vi "Main.vi"(11 "Module Admin":refnum<class "Delacor_lib_QMH_Module Admin.lvclass">) -> ()   [LabVIEW 2014, in "get_data_mapper.lvlib"]
doc: "This template is based off of the Queued Message Handler design pattern and the Queued Message Handler project template that ships with LabVIEW.\n\nThe main difference is that the queue is private to this module and communication between modules is performed via Broadcast and Request events.\n\nRequest events are wrapped in public API methods and are handled in the Event Handling Loop (EHL) of this VI. Any module can register for Broadcast events sent by this module. The EHL generates messages based on user interface actions.\n\nThe Message Handling Loop (MHL) processes messages generated by the EHL, or by other messages. The messages are string values, so new messages can be added easily to the Message Cases case structure in the MHL. Each message cluster can also provide an optional value for Message Data, which is a variant that can be converted to whatever message-specific data is required.\n_____\nBased on DQMH Project Template 6.0.0.91."
uses:
  get_data_mapper.lvlib
  <vilib>/Delacor/Delacor QMH/Libraries/Module Admin_class/Delacor_lib_QMH_Module Admin.lvclass
  Module Data--cluster.ctl
  <vilib>/Delacor/Delacor QMH/Libraries/Message Queue_class/Delacor_lib_QMH_Message Queue.lvclass/Delacor_lib_QMH_Message Queue.ctl
  Stop Argument--cluster.ctl
  <vilib>/Delacor/Delacor QMH/Libraries/Module Admin_class/Delacor_lib_QMH_Module Admin.lvclass/Delacor_lib_QMH_Module Admin.ctl
  <vilib>/Utility/miscctls.llb/LVPointTypeDef.ctl
  <vilib>/Delacor/Delacor QMH/Libraries/Message Queue_class/Delacor_lib_QMH_Enqueue Message (Single).vi
  <vilib>/Delacor/Delacor QMH/Libraries/Module Admin_class/Delacor_lib_QMH_Get External Launch.vi
  <vilib>/Utility/error.llb/Error Cluster From Error Code.vi
  <vilib>/ErrorRing/Error Ring.xnode
  <vilib>/Delacor/Delacor QMH/Libraries/Message Queue_class/Delacor_lib_QMH_Message Queue.lvclass
panel:
  out "Data names":string[](array[string])=["Tc01", "Tc02"]
  in  "Data names Input":string[](array[string])=["Loop_number ", "Error_number", "Error_number_2", "DI_no1", "Flow"]
  in  "Update Names":bool
  out "Data out string":string="{\"Tc01\":1.000000,\"Tc02\":2.000000}"
  in  "Data sources":refnum<k21>[](array[refnum])=["ni.var.psp://my computer/Test Data/testdata1"]
  out "Data Out":dbl[](array[numeric])=[1.0, 2.0]
  out "error out":errorcluster
  out "Status":string="Initial Message"
  in  "Simulate MHL Error":bool
  in  "Simulate EHL Error":bool
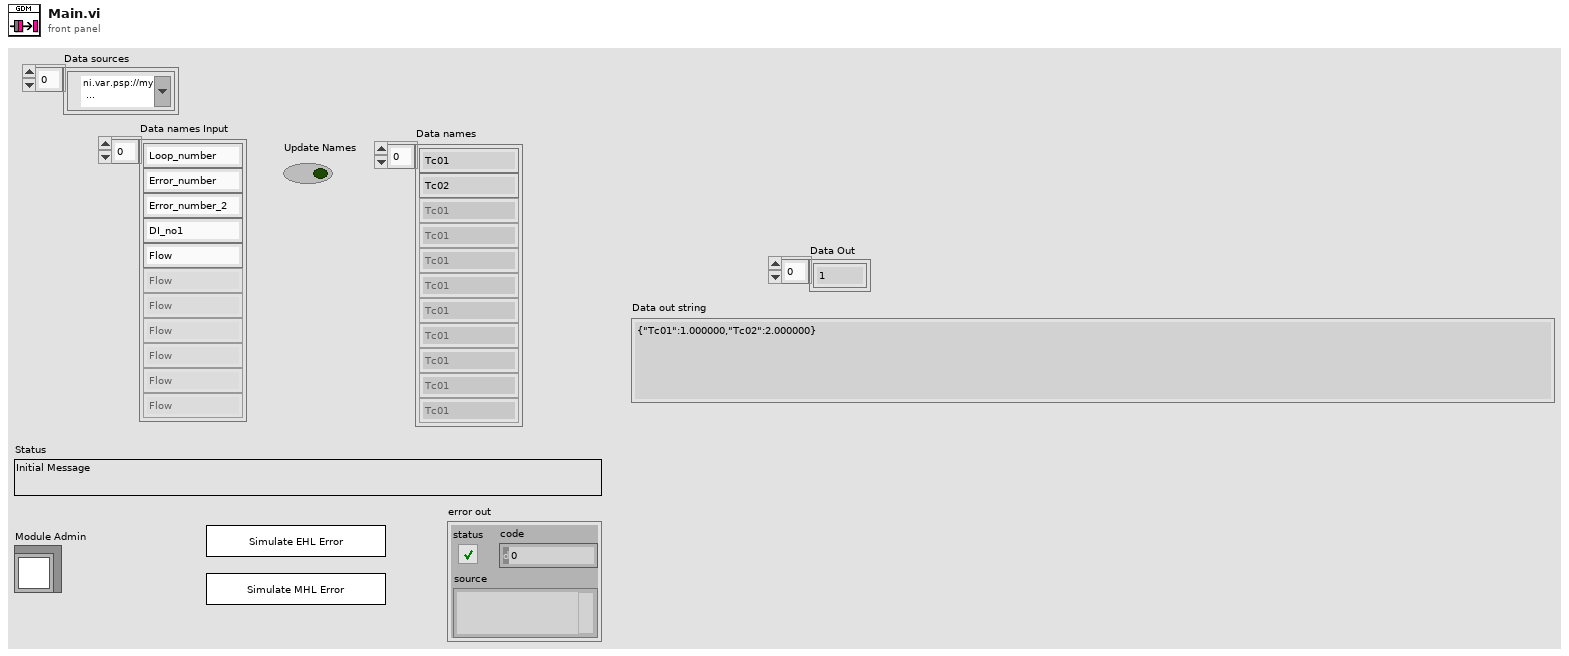
[diagram p1: front panel]
types:
  T1 = typedef "get_data_mapper.lvlib/Request Events--cluster.ctl" = cluster{"Stop Module":refnum<user-event>, "Show Panel":refnum<user-event>, "Hide Panel":refnum<user-event>, "Get Module Execution Status":refnum<user-event>, "Show Diagram":refnum<user-event>}
  T2 = typedef "get_data_mapper.lvlib/Module Data--cluster.ctl" = cluster{"Status":string, "Data sources":refnum<k21>[], "Data Names":string[], "Host name or address":string, "Remote port":u16, "Local port":u16, "Key":string, "connection ID":refnum<k16>}
  T3 = enum32{"invalid lock state", "Not Locked", "Locked (No Password)", "Password-protected"}
  T4 = typedef "get_data_mapper.lvlib/Stop Argument--cluster.ctl" = cluster{"Origin":string, "Exit via Stop Module Req?":bool, "Wait for Module to stop?":bool}
  T5 = typedef "LVPointTypeDef.ctl" = cluster{"Horizontal":i16, "Vertical":i16}
  T6 = enum32{"Invalid", "Standard", "Closed", "Hidden", "Minimized", "Maximized"}
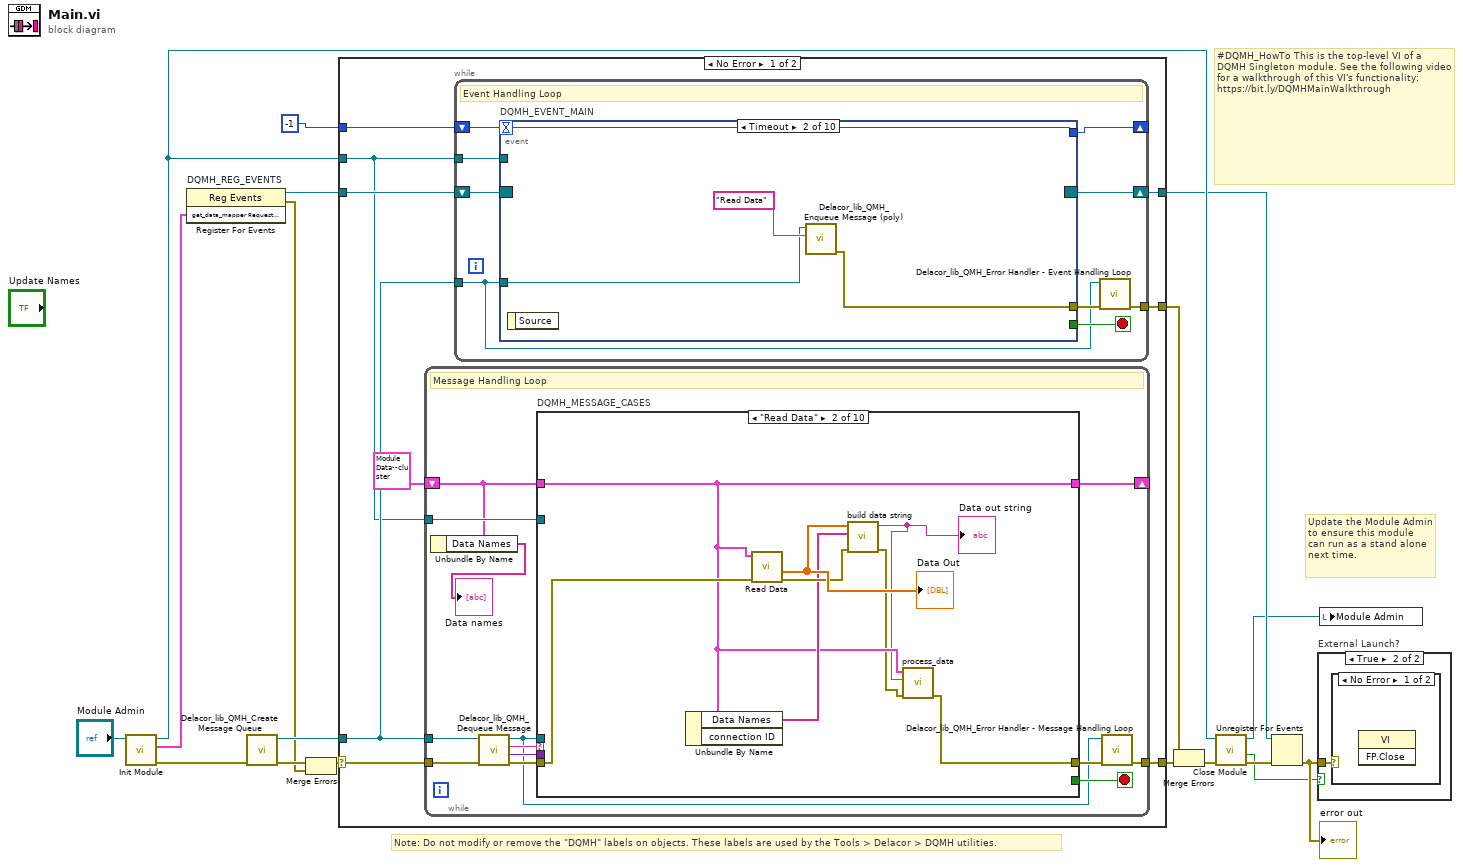
[diagram p0: block diagram]
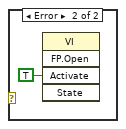
[diagram p3: hidden frame]
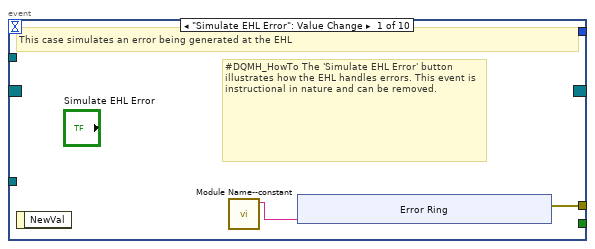
[diagram p4: hidden frame]
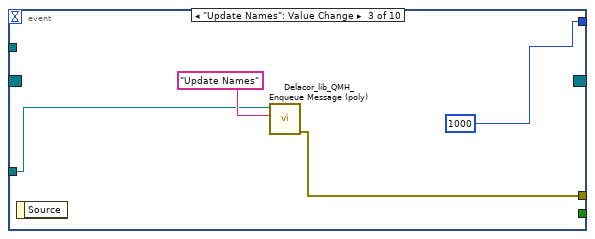
[diagram p5: hidden frame]
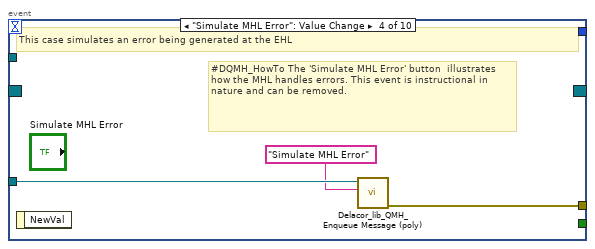
[diagram p6: hidden frame]
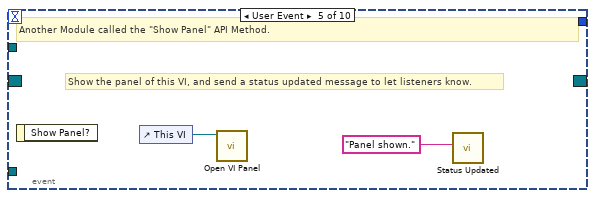
[diagram p7: hidden frame]
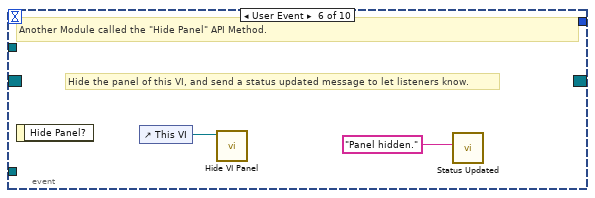
[diagram p8: hidden frame]
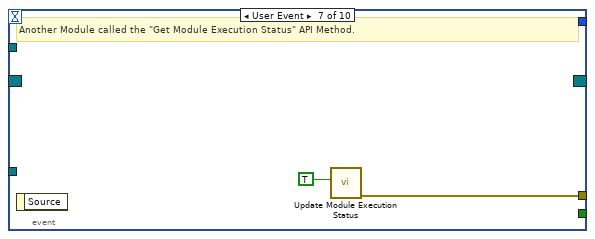
[diagram p9: hidden frame]
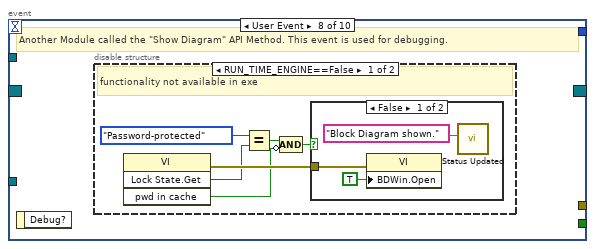
[diagram p10: hidden frame]
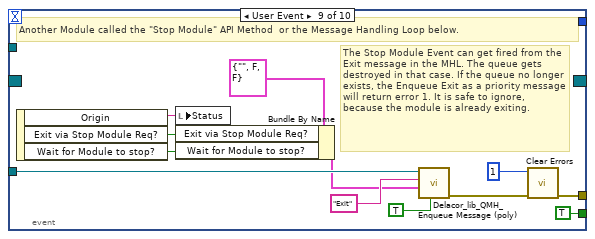
[diagram p13: hidden frame]
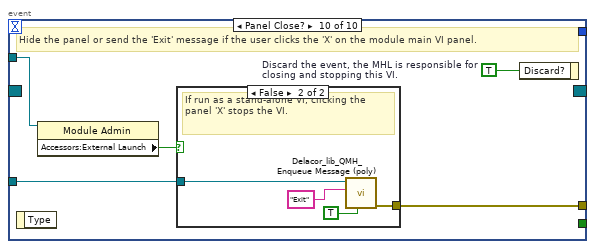
[diagram p14: hidden frame]
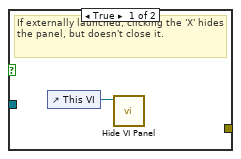
[diagram p15: hidden frame]
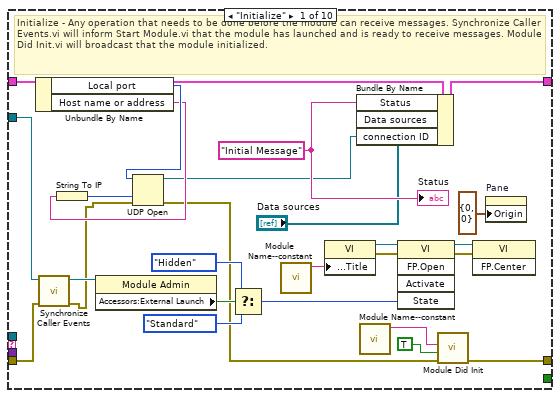
[diagram p16: hidden frame]
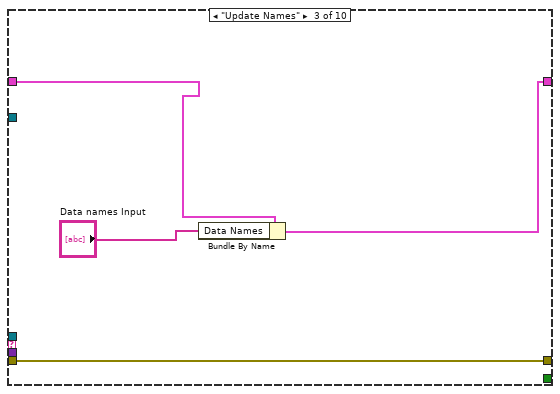
[diagram p17: hidden frame]
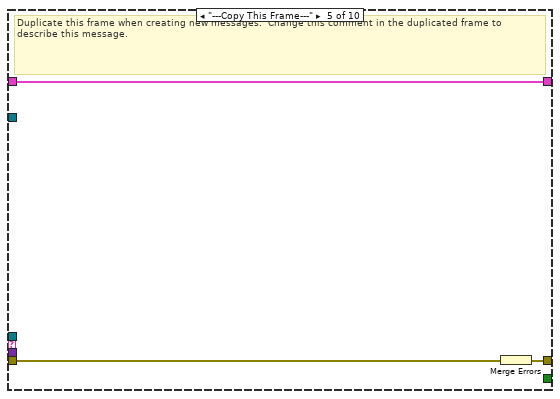
[diagram p19: hidden frame]
diagram:
  # "#DQMH_HowTo This is the top-level VI of a DQMH Singleton module. See the following video for a walkthrough of this VI's functionality: https://bit.ly/DQMHMainWalkthrough"
  # "Note: Do not modify or remove the \"DQMH\" labels on objects. These labels are used by the Tools > Delacor > DQMH utilities."
  # "Update the Module Admin to ensure this module can run as a stand alone next time."
  n1 = call "Init Module.vi"("Singleton Module Admin in"="Module Admin") -> ("error out"=w17:errorcluster, "get_data_mapper Request Events"=w7:T1, "Singleton Module Admin out"=w10:refnum<class "Delacor_lib_QMH_Module Admin.lvclass">)  [unwired: 8 in]
  n2 = register-events "DQMH_REG_EVENTS"(w7) -> (reference out=w8:refnum<event-registration>, error out=w1:errorcluster)  [unwired: 2 in]
  n3 = call <vilib>:"Delacor_lib_QMH_Create Message Queue.vi"("error in"=w17) -> ("error out"=w12:errorcluster, "Message Queue"=w6:refnum<class "Delacor_lib_QMH_Message Queue.lvclass">)  [unwired: 9 in]
  n4 = Merge Errors(w12, w1) -> (w11:errorcluster)
  n5 = case shown="No Error" w11 {
    selector: w11 -> [w25 w211]
    tunnel: [w27 w210] -> w18
    tunnel: [w24 w216] -> w9
    tunnel: w8 -> [w22 w216]
    tunnel: w6 -> [w21 w209]
    tunnel: [w26 _] -> w15
    tunnel: w10 -> [w20 w212]
    tunnel: -1 -> [w19 _]
    frame No Error {
      n6 = while {
        tunnel: w21 -> [w98]
        shift-right: [w102] -> _
        shift-left: T2 {"Status"="", "Data sources"=[], "Data Names"=[], "Host name or address"="localhost", "Remote port"=35536, "Local port"=35535, "Key"="0123456789abcdef", "connection ID"=refnum} ("Data Cluster") -> [w95]
        tunnel: w25 -> [w105]
        tunnel: [w103] -> w27
        tunnel: w20 -> [w96]
        stop <- w101 stop-if-true
        # "Message Handling Loop"
        n7 = Unbundle By Name(w95) -> ("Data Names"=→"Data names":string[])
        n8 = call-dynamic "Delacor_lib_QMH_Dequeue Message.vi"("error in"=w105, "Message Queue in"=w98) -> ("error out"=w104:errorcluster, "Message Data"=w99:variant, "Message"=w100:string, "Message Queue out"=w97:refnum<class "Delacor_lib_QMH_Message Queue.lvclass">)  [unwired: 6 in]
        n9 = case "DQMH_MESSAGE_CASES" shown="\"Read Data\"" w100 {
          selector: w100 -> [_ _ _ _ _ _ _ _ _ w196]
          tunnel: w97 -> [_ _ _ _ _ _ _ w166 w188 _]
          tunnel: w104 -> [w130 w140 w144 w146 w149 w151 w156 w173 w194 w198]
          tunnel: [w129 w133 w144 w146 w148 w151 w155 w169 w191 w199] -> w106
          tunnel: w95 -> [w113 w136 w143 w145 w147 w150 w153 w168 w187 w197]
          tunnel: [w120 w136 w142 w145 w147 w150 w153 w168 w187 w197] -> w102
          tunnel: [_ _ _ _ _ _ _ _ w186 _] -> w101
          tunnel: w99 -> [_ _ _ _ _ _ _ w167 w185 _]
          tunnel: w96 -> [w121 _ _ _ _ _ _ w165 w180 _]
          frame "Initialize" {
            w116 = "Initial Message" ("Initial Message")
            # "Initialize - Any operation that needs to be done before the module can receive messages. Synchronize Caller Events.vi will inform Start Module.vi that the module has launched and is ready to receive messages. Module Did Init.vi will broadcast that the module initialized."
            n10 = Unbundle By Name(w113) -> ("Local port"=w112:u16, "Host name or address"=w111:string)
            n11 = call "Synchronize Caller Events.vi"("error in (no error)"=w130, "Singleton Module Admin in"=w121) -> ("error out"=w109:errorcluster, "Singleton Module Admin out"=w117:refnum<class "Delacor_lib_QMH_Module Admin.lvclass">)  [unwired: 8 in]
            n12 = String To IP(1:w111) -> (0:w110:u32)
            n13 = property class="Module Admin"(reference=w117) -> ("Accessors:External Launch"=w125:bool)  [unwired: 1 in, 2 out]
            n14 = UDP Open(7:w110, 8:w109, 11:w112) -> (port=w107:refnum<k16>, 0:w108:errorcluster)  [unwired: 2 in, 1 out]
            n15 = Select(t=T6."Hidden" ("State"), s=w125, f=T6."Standard" ("State")) -> (s? t:f=w122:T6)
            n16 = call "Module Name--constant.vi"() -> ("Module Name"=w128:string)  [unwired: 11 in]
            n17 = property class="VI"("Front Panel.Title"=w128) -> (reference out=w127:refnum<vi>, error out=w132:errorcluster)  [unwired: 2 in]
            n18 = Bundle By Name(cluster=w113, "Status"=w116, "Data sources"="Data sources", "connection ID"=w107) -> (w120:T2)
            n19 = call "Module Name--constant.vi"() -> ("Module Name"=w118:string)  [unwired: 11 in]
            n20 = invoke class="VI" method="FP.Open"(reference=w127, error in=w132, "State"=w122) -> (reference out=w126:refnum<vi>, error out=w131:errorcluster)  [unwired: 2 in, 3 out]
            n21 = call "Module Did Init.vi"("error in (no error)"=w108, "Initialized?"=TRUE, "Origin"=w118) -> ("error out"=w129:errorcluster)  [unwired: 8 in]
            n22 = invoke class="VI" method="FP.Center"(reference=w126, error in=w131) -> ()  [unwired: 1 in, 3 out]
            n23 = property on="Pane" class="Pane"("Origin"=T5 {"Horizontal"=0, "Vertical"=0}) -> ()  [unwired: 2 in, 2 out]
            "Status" <- w116
          }
          frame "Read Data" {
            n24 = Unbundle By Name(w136) -> ("Data Names"=w137:string[])  [unwired: 1 out]
            n25 = call "Read Data.vi"("error in (no error)"=w140, "Data Cluster"=w136) -> ("error in (no error) 2"=w138:errorcluster, "Array"=w139:dbl[])  [unwired: 8 in]
            "Data Out" <- w139
            n26 = call "build data string.vi"("Data in"=w139, "String in"=w137, "error constant 2"=w138) -> ("Data out"=w135:string, "error constant"=w134:errorcluster)  [unwired: 6 in]
            "Data out string" <- w135
            n27 = call "process_data.vi"("Error in"=w134, "JSON Payload"=w135, "Data Cluster in"=w136) -> ("Error out"=w133:errorcluster)  [unwired: 7 in, 1 out]
          }
          frame "Update Names" {
            n28 = Bundle By Name(cluster=w143, "Data Names"="Data names Input") -> (w142:T2)
          }
          frame "---Module Specific---" {
            # "Separator -- The following cases handle messages specific to this Module."
          }
          frame "---Copy This Frame---" {
            # "Duplicate this frame when creating new messages.  Change this comment in the duplicated frame to describe this message."
            n29 = Merge Errors(w149) -> (w148:errorcluster)
          }
          frame "---Exit and Error Handling---" {
            # "Separator - The following cases handle errors and exit messages."
          }
          frame "Simulate MHL Error" {
            # "#DQMH_HowTo The 'Simulate MHL Error' button  illustrates how the MHL handles errors. This event is instructional in nature and can be removed."
            # "Simulate an error occurring at the MHL"
            n30 = call "Module Name--constant.vi"() -> ("Module Name"=w152:string)  [unwired: 11 in]
            n31 = xnode "Error Ring"("parameter 0"=w152) -> ("error out"=w154:errorcluster)
            n32 = Merge Errors(w156, w154) -> (w155:errorcluster)
          }
          frame "Error" {
            # "#CodeRecommended - If you ever change the name of this \"Error\" message, you'll need to update the name in the Check Loop Error.vi as well."
            # "#CodeRecommended - If the module is running in standalone mode (External Launch = FALSE), this code will pop up an error dialog and call the 'Exit' message if an error occurs. Add more fine-grained error handling here."
            # "Error - Check the error message data and respond accordingly. This message is sent by the \"Error Handler\" VIs at the end of each loop in this application."
            n33 = property class="Module Admin"(reference=w165) -> ("Accessors:External Launch"=w164:bool)  [unwired: 1 in, 2 out]
            n34 = Variant To Data(error in=w173, type=errorcluster {"status"=FALSE, "code"=0, "source"=""} ("error constant"), Variant=w167) -> (data=w174:errorcluster, error out=w171:errorcluster)
            n35 = call "Error Reported.vi"("Error"=w174) -> ()  [unwired: 10 in, 1 out]
            n36 = case shown="False" w164 {
              tunnel: [w179 _] -> w170
              tunnel: w166 -> [w177 _]
              tunnel: w174 -> [w178 _]
              frame False {
                # "If the module is running standalone, then pop up an error dialog and call the \"Exit\" message."
                n37 = call <vilib>:"Simple Error Handler.vi"("error in (no error)"=w178) -> ()  [unwired: 4 in, 5 out]
                n38 = call-poly <vilib>:"Delacor_lib_QMH_Enqueue Message (poly).vi"("Priority Message? (F)"=TRUE, "Message"="Exit", "Message Queue in"=w177) -> ("error out"=w179:errorcluster)  [unwired: 7 in, 1 out]
              }
              frame True {
                # "If the module was launched externally, calling the Error Reported broadcast VI is the only action performed by the \"Error\" message. The module's caller can then process the error appropriately."
              }
            }
            n39 = Merge Errors(w171, w170) -> (w169:errorcluster)
            n40 = local write "error out"(w169) -> ()
          }
          frame "Exit" {
            w184 = 91  # 91: not all Exit messages will have an argument
            w186 = TRUE  # Stop the VI
            # "Release the message queue reference"
            # "#CodeNeeded - Add any required cleanup code here"
            # "Exit - Exit the application."
            n41 = Variant To Data(error in=w194, type=T4 {"Origin"="", "Exit via Stop Module Req?"=FALSE, "Wait for Module to stop?"=FALSE} ("Stop Argument"), Variant=w185) -> (data=w182:T4, error out=w190:errorcluster)
            n42 = call <vilib>:"Clear Errors.vi"("error in (no error)"=w190, "specific error code to clear (0: all)"=w184) -> ("error out"=w193:errorcluster)  [unwired: 4 in, 1 out]
            n43 = control-ref of="This VI"() -> (w181:refnum<vi>)
            n44 = call-dynamic "Delacor_lib_QMH_Release Message Queue.vi"("error in"=w193, "Message Queue"=w188) -> ("error out"=w192:errorcluster)  [unwired: 9 in]
            n45 = call "Handle Exit.vi"("Stop Argument"=w182, "Admin in"=w180, "VI reference"=w181) -> ("error out"=w189:errorcluster)  [unwired: 7 in, 1 out]
            n46 = Merge Errors(w192, w189) -> (w191:errorcluster)
          }
          frame Default {
            # "'Default' case only runs if there is a message that isn't defined in any of the other cases.  Output a programming error."
            n47 = call "Module Name--constant.vi"() -> ("Module Name"=w195:string)  [unwired: 11 in]
            n48 = xnode "Error Ring"("parameter 0"=w196, "parameter 1"=w195) -> ("error out"=w200:errorcluster)
            n49 = Merge Errors(w198, w200) -> (w199:errorcluster)
          }
        }
        n50 = call-dynamic "Delacor_lib_QMH_Error Handler - Message Handling Loop.vi"("error in"=w106, "Message Queue in"=w97) -> ("dup error in"=w103:errorcluster)  [unwired: 8 in, 1 out]
      }
      n51 = while {
        tunnel: w21 -> [w30]
        shift-right: [w33] -> w24
        shift-left: w22 -> [w34]
        tunnel: [w35] -> w26
        tunnel: w20 -> [w31]
        shift-right: [w28] -> _
        shift-left: w19 -> [w29]
        stop <- w32 stop-if-true
        # "Event Handling Loop"
        n52 = event "DQMH_EVENT_MAIN" shown="[1] Timeout" {
          selector: w34 -> [_ _ _ _ _ _ _ _ _ _]
          dyn-events: [_ _ _ _ _ _ _ _ _ _] -> w33
          timeout: w29 -> [_ w46 _ _ _ _ _ _ _ _]
          tunnel: [_ _ _ _ _ _ _ _ TRUE ("Discard?") _] -> w32
          tunnel: w30 -> [_ w48 w52 w55 _ _ _ _ w79 w86]
          tunnel: [w38 w47 w51 w56 _ _ w62 _ w82 w88] -> w36
          tunnel: w31 -> [_ _ _ _ _ _ _ _ _ w85]
          tunnel: [_ w46 1000 _ _ _ _ _ _ _] -> w28
          event "Simulate EHL Error": Value Change {
            # "#DQMH_HowTo The 'Simulate EHL Error' button  illustrates how the EHL handles errors. This event is instructional in nature and can be removed."
            # "This case simulates an error being generated at the EHL"
            n53 = event-data() -> ()  [unwired: 1 in, 1 out]
            n54 = call "Module Name--constant.vi"() -> ("Module Name"=w37:string)  [unwired: 11 in]
            n55 = xnode "Error Ring"("parameter 0"=w37) -> ("error out"=w38:errorcluster)
          }
          event Timeout {
            n56 = event-data() -> ()  [unwired: 1 in, 1 out]
            n57 = call-poly <vilib>:"Delacor_lib_QMH_Enqueue Message (poly).vi"("Message"="Read Data", "Message Queue in"=w48) -> ("error out"=w47:errorcluster)  [unwired: 8 in, 1 out]
          }
          event "Update Names": Value Change {
            n58 = event-data() -> ()  [unwired: 1 in, 1 out]
            n59 = call-poly <vilib>:"Delacor_lib_QMH_Enqueue Message (poly).vi"("Message"="Update Names", "Message Queue in"=w52) -> ("error out"=w51:errorcluster)  [unwired: 8 in, 1 out]
          }
          event "Simulate MHL Error": Value Change {
            # "#DQMH_HowTo The 'Simulate MHL Error' button  illustrates how the MHL handles errors. This event is instructional in nature and can be removed."
            # "This case simulates an error being generated at the EHL"
            n60 = event-data() -> ()  [unwired: 1 in, 1 out]
            n61 = call-poly <vilib>:"Delacor_lib_QMH_Enqueue Message (poly).vi"("Message"="Simulate MHL Error", "Message Queue in"=w55) -> ("error out"=w56:errorcluster)  [unwired: 8 in, 1 out]
          }
          event User Event {
            # "Show the panel of this VI, and send a status updated message to let listeners know."
            # "Another Module called the \"Show Panel\" API Method."
            n62 = event-data() -> ()  [unwired: 1 in, 1 out]
            n63 = control-ref of="This VI"() -> (w58:refnum<vi>)
            n64 = call "Open VI Panel.vi"("VI"=w58) -> ()  [unwired: 10 in, 1 out]
            n65 = call "Status Updated.vi"("Status"="Panel shown." ("format string")) -> ()  [unwired: 10 in, 1 out]
          }
          event User Event {
            # "Hide the panel of this VI, and send a status updated message to let listeners know."
            # "Another Module called the \"Hide Panel\" API Method."
            n66 = event-data() -> ()  [unwired: 1 in, 1 out]
            n67 = control-ref of="This VI"() -> (w60:refnum<vi>)
            n68 = call "Hide VI Panel.vi"("VI"=w60) -> ()  [unwired: 10 in, 1 out]
            n69 = call "Status Updated.vi"("Status"="Panel hidden." ("format string")) -> ()  [unwired: 10 in, 1 out]
          }
          event User Event {
            # "Another Module called the \"Get Module Execution Status\" API Method."
            n70 = event-data() -> ()  [unwired: 1 in, 1 out]
            n71 = call "Update Module Execution Status.vi"("Running?"=TRUE) -> ("error out"=w62:errorcluster)  [unwired: 10 in]
          }
          event User Event {
            # "Another Module called the \"Show Diagram\" API Method. This event is used for debugging."
            n72 = event-data() -> ()  [unwired: 1 in, 1 out]
            n73 = disable-structure shown="RUN_TIME_ENGINE==False" {
              frame condition #0 (active) {
                # "functionality not available in exe"
                n74 = invoke class="VI" method="Lock State.Get"() -> (error out=w68:errorcluster, "Get Lock State"=w67:T3, "pwd in cache"=w64:bool)  [unwired: 4 in, 1 out]
                n75 = Equal?(x=T3."Password-protected", y=w67) -> (x = y?=w65:bool)
                n76 = Compound Arithmetic op=AND(w65, invert w64) -> (w63:bool)
                n77 = case shown="False" w63 {
                  tunnel: w68 -> [w71 _]
                  frame False {
                    n78 = property class="VI"(error in=w71, "BDWin.Open"=TRUE ("Block Diagram Window:Open")) -> ()  [unwired: 1 in, 2 out]
                    n79 = call "Status Updated.vi"("Status"="Block Diagram shown." ("format string")) -> ()  [unwired: 10 in, 1 out]
                  }
                  frame True {
                    # "Password-protected VI, and the password is not in the cache. Do not show the diagram."
                  }
                }
              }
              frame condition #1 {
              }
            }
          }
          event User Event {
            # "The Stop Module Event can get fired from the Exit message in the MHL. The queue gets destroyed in that case. If the queue no longer exists, the Enqueue Exit as a priority message will return error 1. It is safe to ignore, because the module is already exiting."
            # "Another Module called the \"Stop Module\" API Method  or the Message Handling Loop below."
            n80 = event-data() -> ("Origin"=w78:string, "Exit via Stop Module Req?"=w74:bool, "Wait for Module to stop?"=w73:bool)  [unwired: 1 in]
            n81 = local write "Status"(w78) -> ()
            n82 = Bundle By Name(cluster=T4 {"Origin"="", "Exit via Stop Module Req?"=FALSE, "Wait for Module to stop?"=FALSE} ("Stop Argument"), "Exit via Stop Module Req?"=w74, "Wait for Module to stop?"=w73) -> (w72:T4)
            n83 = call-poly <vilib>:"Delacor_lib_QMH_Enqueue Message (poly).vi"("Priority Message? (F)"=TRUE, "Message Data"=w72, "Message"="Exit", "Message Queue in"=w79) -> ("error out"=w83:errorcluster)  [unwired: 6 in, 1 out]
            n84 = call <vilib>:"Clear Errors.vi"("error in (no error)"=w83, "specific error code to clear (0: all)"=1) -> ("error out"=w82:errorcluster)  [unwired: 4 in, 1 out]
          }
          event Panel Close? {
            w87 = TRUE  # Discard the event, the MHL is responsible for closing and stopping this VI.
            # "Hide the panel or send the 'Exit' message if the user clicks the 'X' on the module main VI panel."
            n85 = event-data() -> ()  [unwired: 1 in, 1 out]
            n86 = property class="Module Admin"(reference=w85) -> ("Accessors:External Launch"=w84:bool)  [unwired: 1 in, 2 out]
            n87 = case shown="False" w84 {
              tunnel: w86 -> [_ w92]
              tunnel: [_ w93] -> w88
              frame True {
                # "If externally launched, clicking the 'X' hides the panel, but doesn't close it."
                n88 = control-ref of="This VI"() -> (w89:refnum<vi>)
                n89 = call "Hide VI Panel.vi"("VI"=w89) -> ()  [unwired: 10 in, 1 out]
              }
              frame False {
                # "If run as a stand-alone VI, clicking the panel 'X' stops the VI."
                n90 = call-poly <vilib>:"Delacor_lib_QMH_Enqueue Message (poly).vi"("Priority Message? (F)"=TRUE, "Message"="Exit", "Message Queue in"=w92) -> ("error out"=w93:errorcluster)  [unwired: 7 in, 1 out]
              }
            }
            n91 = event-data("Discard?"=w87) -> ()  [unwired: 1 in, 1 out]
          }
        }
        n92 = call-dynamic "Delacor_lib_QMH_Error Handler - Event Handling Loop.vi"("error in"=w36, "Message Queue in"=w30) -> ("dup error in"=w35:errorcluster)  [unwired: 8 in, 1 out]
      }
    }
    frame Error {
      # "Synchronize Caller Events.vi will inform Start Module.vi that the module has launched and will let the code calling Start Module.vi register for broadcasts and would permit the caller receive the broadcast that an error occurred at launch time."
      n93 = call-dynamic "Delacor_lib_QMH_Release Message Queue.vi"("error in"=w211, "Message Queue"=w209) -> ("error out"=w210:errorcluster)  [unwired: 9 in]
      n94 = call "Synchronize Caller Events.vi"("Singleton Module Admin in"=w212) -> ("error out"=w217:errorcluster)  [unwired: 9 in, 1 out]
      n95 = call "Module Name--constant.vi"() -> ("Module Name"=w215:string)  [unwired: 11 in]
      n96 = Format Into String(format string="An error occurred during initialization. %s is no longer running.", w215) -> (resulting string=w213:string)  [unwired: 2 in, 1 out]
      n97 = Merge Errors(w210, w217) -> (w218:errorcluster)
      n98 = call "Error Reported.vi"("Additional Information"=w213, "Error"=w218) -> ()  [unwired: 9 in, 1 out]
    }
  }
  n99 = Merge Errors(w15, w18) -> (w14:errorcluster)
  n100 = call "Close Module.vi"("error in (no error)"=w14, "Module Admin in"=w10) -> ("error out"=w16:errorcluster, "External Launch"=w3:bool, "Module Admin out"=w4:refnum<class "Delacor_lib_QMH_Module Admin.lvclass">)  [unwired: 7 in]
  n101 = Unregister For Events(event registration refnum=w9, error in=w16) -> (error out=w13:errorcluster)
  "error out" <- w13
  n102 = case "External Launch?" shown="True" w3 {
    tunnel: w13 -> [_ w219]
    frame False {
    }
    frame True {
      n103 = case shown="No Error" w219 {
        frame No Error {
          n104 = invoke class="VI" method="FP.Close"() -> ()  [unwired: 3 in, 3 out]
        }
        frame Error {
          n105 = invoke class="VI" method="FP.Open"("Activate"=TRUE ("Activate?")) -> ()  [unwired: 4 in, 5 out]
        }
      }
    }
  }
  n106 = local write "Module Admin"(w4) -> ()
